vi "Create 1D Table.vi"(8 "formatted values":string[](array[string]), 11 "table name":string) -> (3 "table":string)   [LabVIEW 2013, in "infolib.lvlib"]
uses:
  infolib.lvlib
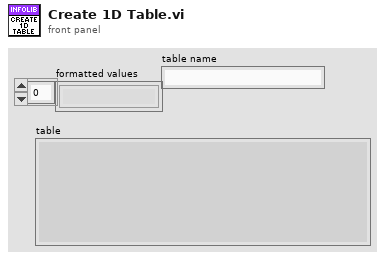
[diagram p1: front panel]
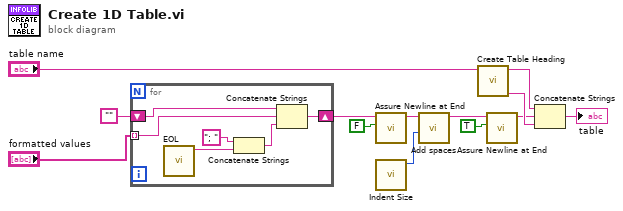
[diagram p0: block diagram]
diagram:
  n1 = for {
    tunnel: "formatted values" -> [w15] mode=indexing
    shift-right: [w14] -> w5
    shift-left: "" -> [w19]
    n2 = call "EOL.vi"() -> ("eol"=w18:string)  [unwired: 11 in]
    n3 = Concatenate Strings("; " ("delimiter (Tab)"), w18) -> (w16:string)
    n4 = Concatenate Strings(w19, w15, w16) -> (w14:string)
  }
  n5 = call "Assure Newline at End.vi"("Set End Of Line (F)"=FALSE, "string"=w5) -> ("string out"=w6:string)  [unwired: 9 in]
  n6 = call "Indent Size.vi"() -> ("indent size"=w7:i32)  [unwired: 11 in]
  n7 = call "Add spaces.vi"("spaces no"=w7, "input string"=w6) -> ("result string"=w3:string)  [unwired: 9 in]
  n8 = call "Create Table Heading.vi"("table name"="table name") -> ("table end"=w9:string, "table start"=w10:string)  [unwired: 9 in]
  n9 = call "Assure Newline at End.vi"("Set End Of Line (F)"=TRUE, "string"=w3) -> ("string out"=w2:string)  [unwired: 9 in]
  n10 = Concatenate Strings(w10, w2, w9) -> (→"table":string)
